vi "Preferences.vi"(11 "Preferences in":T1) -> (0 "error out":errorcluster, 3 "Preferences out":T1)   [LabVIEW 2020]
uses:
  Preferences.ctl
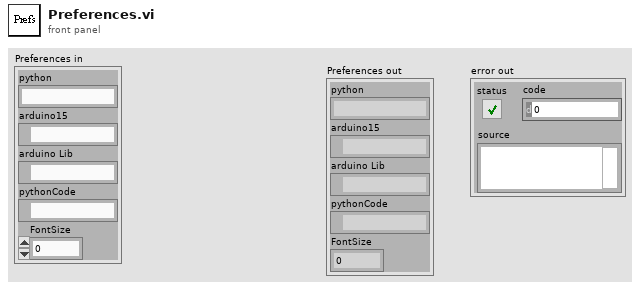
[diagram p1: front panel]
types:
  T1 = typedef "Preferences.ctl" = cluster{"python":string, "arduino15":path, "arduino Lib":path, "pythonCode":path, "FontSize":u8}
  T2 = cluster{"python":string, "arduino15":string, "arduino Lib":string, "PythonCodePath":string, "FontSize":string}
  T3 = cluster{"[0]":string, "[1]":string, "[2]":string, "[3]":string, "[4]":string}
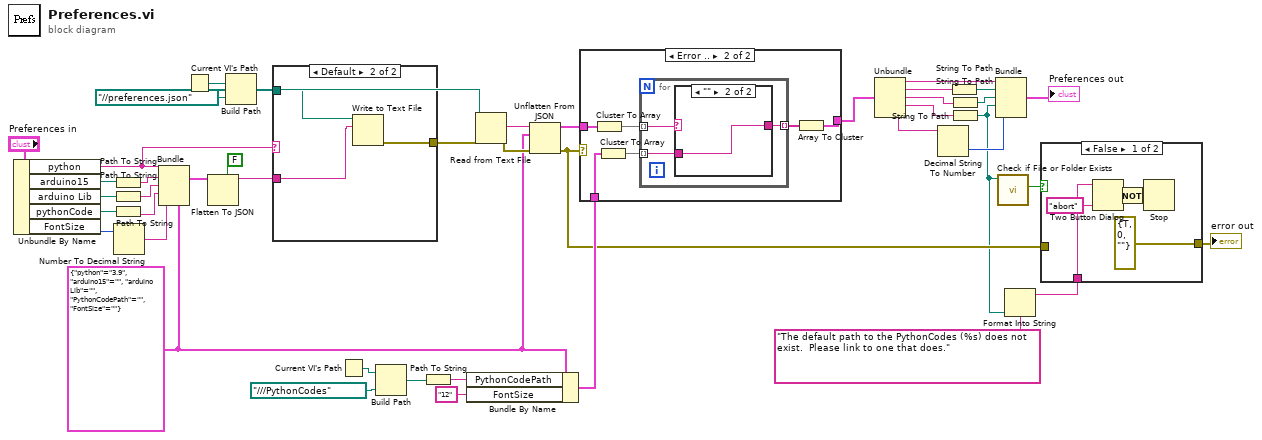
[diagram p0: block diagram]
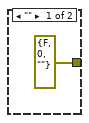
[diagram p3: hidden frame]
diagram:
  w14 = T2 {"python"="3.9", "arduino15"="", "arduino Lib"="", "PythonCodePath"="", "FontSize"=""} ("Preferences")
  n1 = Unbundle By Name("Preferences in") -> ("python"=w36:string, "arduino15"=w35:path, "arduino Lib"=w34:path, "pythonCode"=w26:path, "FontSize"=w9:u8)
  n2 = Path To String(path=w35) -> (string=w29:string)
  n3 = Path To String(path=w34) -> (string=w28:string)
  n4 = Path To String(path=w26) -> (string=w27:string)
  n5 = Number To Decimal String(number=w9) -> (decimal integer string=w8:string)  [unwired: 1 in]
  n6 = Bundle(cluster=w14, "python"=w36, "arduino15"=w29, "arduino Lib"=w28, "PythonCodePath"=w27, "FontSize"=w8) -> (w32:T2)
  n7 = Current VI's Path() -> (path=w39:path)
  n8 = Flatten To JSON(enable LabVIEW extensions? (T)=FALSE, anything=w32) -> (JSON string=w31:string)  [unwired: 1 in, 1 out]
  n9 = Build Path(base path=w39, name or relative path=path "../../preferences.json") -> (appended path=w30:path)
  n10 = case shown="Default" w36 {
    tunnel: [errorcluster {"status"=FALSE, "code"=0, "source"=""} ("error out") w47] -> w40
    tunnel: w30 -> [_ w46]
    tunnel: w31 -> [_ w45]
    frame "" {
    }
    frame Default {
      n11 = Write to Text File(file (use dialog)=w46, text=w45) -> (error out=w47:errorcluster)  [unwired: 2 in, 2 out]
    }
  }
  n12 = Current VI's Path() -> (path=w17:path)
  n13 = Build Path(base path=w17, name or relative path=path "../../../PythonCodes") -> (appended path=w7:path)
  n14 = Path To String(path=w7) -> (string=w15:string)
  n15 = Bundle By Name(cluster=w14, "PythonCodePath"=w15, "FontSize"="12") -> (w13:T2)
  n16 = Read from Text File(file (use dialog)=w30, error in=w40) -> (text=w43:string, error out=w41:errorcluster)  [unwired: 2 in, 2 out]
  n17 = Unflatten From JSON(JSON string=w43, type and defaults=w14, error in (no error)=w41) -> (value=w42:T2, error out=w5:errorcluster)  [unwired: 4 in]
  n18 = case shown="Error .." w5 {
    tunnel: w42 -> [w48 w54]
    tunnel: [w48 w51] -> w19
    tunnel: w13 -> [_ w50]
    frame No Error {
    }
    frame Error {
      n19 = Cluster To Array(cluster=w54) -> (array=w53:string[])
      n20 = Cluster To Array(cluster=w50) -> (array=w49:string[])
      n21 = for {
        tunnel: w53 -> [w57] mode=indexing
        tunnel: [w56] -> w52 mode=indexing
        tunnel: w49 -> [w55] mode=indexing
        n22 = case shown="\"\"" w57 {
          selector: w57 -> [w58 _]
          tunnel: [w58 w59] -> w56
          tunnel: w55 -> [_ w59]
          frame Default {
          }
          frame "" {
          }
        }
      }
      n23 = Array To Cluster(array=w52) -> (cluster=w51:T3)
    }
  }
  n24 = Unbundle(w19) -> ("[0]"=w23:string, "[1]"=w20:string, "[2]"=w21:string, "[3]"=w25:string, "[4]"=w11:string)
  n25 = Decimal String To Number(string=w11) -> (number=w10:i32)  [unwired: 2 in, 1 out]
  n26 = String To Path(string=w20) -> (path=w24:path)
  n27 = String To Path(string=w21) -> (path=w22:path)
  n28 = String To Path(string=w25) -> (path=w2:path)
  n29 = Bundle("[0]"=w23, w24, w22, w2, w10) -> (→"Preferences out":cluster{"[0]":string, path, path, path, i32})  [unwired: 1 in]
  n30 = call <vilib>:"Check if File or Folder Exists.vi"("path"=w2) -> ("file or folder exists?"=w6:bool)  [unwired: 8 in, 2 out]
  n31 = Format Into String(format string="The default path to the PythonCodes (%s) does not exist.  Please link to one that does." ("message"), w2) -> (resulting string=w1:string)  [unwired: 2 in, 1 out]
  n32 = case shown="False" w6 {
    tunnel: w1 -> [w64 _]
    tunnel: w5 -> [_ w65]
    tunnel: [errorcluster {"status"=TRUE, "code"=0, "source"=""} ("error out") w65] -> w4
    frame False {
      n33 = Two Button Dialog(message=w64, 1:"abort" ("F button name (\"Cancel\")")) -> (T button?=w61:bool)  [unwired: 1 in]
      n34 = Not(x=w61) -> (.not. x?=w60:bool)
      n35 = Stop(stop? (T)=w60) -> ()
    }
    frame True {
    }
  }
  "error out" <- w4
